vi "PosStrikerAnguloAttacker.vi"(8 "AnguloGol":dbl, 9 "atacando contra":bool, 10 "IA State":T1={"our_robots"=[], "enemy_robots"=[], "balls"=[], "geometry"={"line_width"=0, "field_length"=0, "field_width"=0, "boundary_width"=0, "referee_width"=0, "goal_width"=0, "goal_depth"=0, "goal_wall_width"=0, "center_circle_radius"=0, "defense_radius"=0, "defense_stretch"=0, "free_kick_from_defense_dist"=0, "penalty_spot_from_field_line_dist"=0, "penalty_line_from_spot_dist"=0}, "IA Judge"={"stage"="", "command"="", "our_goalie_id"=0.0, "enemy_goalie_id"=0.0, "command enum"=enum."Halt", "Time"=enum."Azul"}, "Received Timestamp"=timestamp(0 s since 1904-01-01), "Events"={"Touch"=FALSE, "Ball out"=FALSE, "id touch"=0.0, "Ball out of \nVision"=FALSE, "Ball inside \nGoalie area"=FALSE, "Robot not responding"=FALSE, "Robots responding status"=[1.0, 1.0, 1.0, 1.0, 1.0, 1.0], "Enemy Ball \nPossession"=FALSE, "Pass State"=FALSE, "id end of pass"=0.0, "Kick"=FALSE, "Id Possession"=0.0}, "Position"=[]}) -> (0 "YdoAttacker 2":dbl, 1 "AttackerPositive?":bool, 2 "theta final":dbl, 3 "XdoAttacker 2":dbl)   [LabVIEW 2016]
uses:
  Core/AI Input.ctl
  Core/AI Robot.ctl
  Intel/Functions Enum.ctl
  Intel/AttackerStates.ctl
  Core/AI Ball.ctl
  Core/Field Size.ctl
  Core/AI Judge.ctl
  Intel/Command Enum.ctl
  Events/Events.ctl
panel:
  in  "valor de theta 3":dbl
  in  "tamanho do intervalo 3":dbl
  in  "inicio do intervalo 3":dbl
  in  "fim do intervalo 3":dbl
  in  "Contador 4":dbl
  in  "Array 3":dbl[](array[numeric])=[0.0, 0.0, 0.0, 0.0, 0.0, 0.0]
  in  "valor de theta 2":dbl
  in  "tamanho do intervalo 2":dbl
  in  "inicio do intervalo 2":dbl
  in  "fim do intervalo 2":dbl
  in  "Contador 3":dbl
  in  "Array 2":dbl[](array[numeric])=[0.0, 0.0, 0.0, 0.0, 0.0, 0.0]
  in  "XdoAttacker":dbl
  in  "YdoAttacker":dbl
  in  "RobôsParaAnalisar":dbl[][](array[numeric])=[[99999.0, 99999.0], [99999.0, 99999.0], [99999.0, 99999.0], [99999.0, 99999.0], [99999.0, 99999.0], [99999.0, 99999.0], [99999.0, 99999.0]]
  in  "Contador":dbl
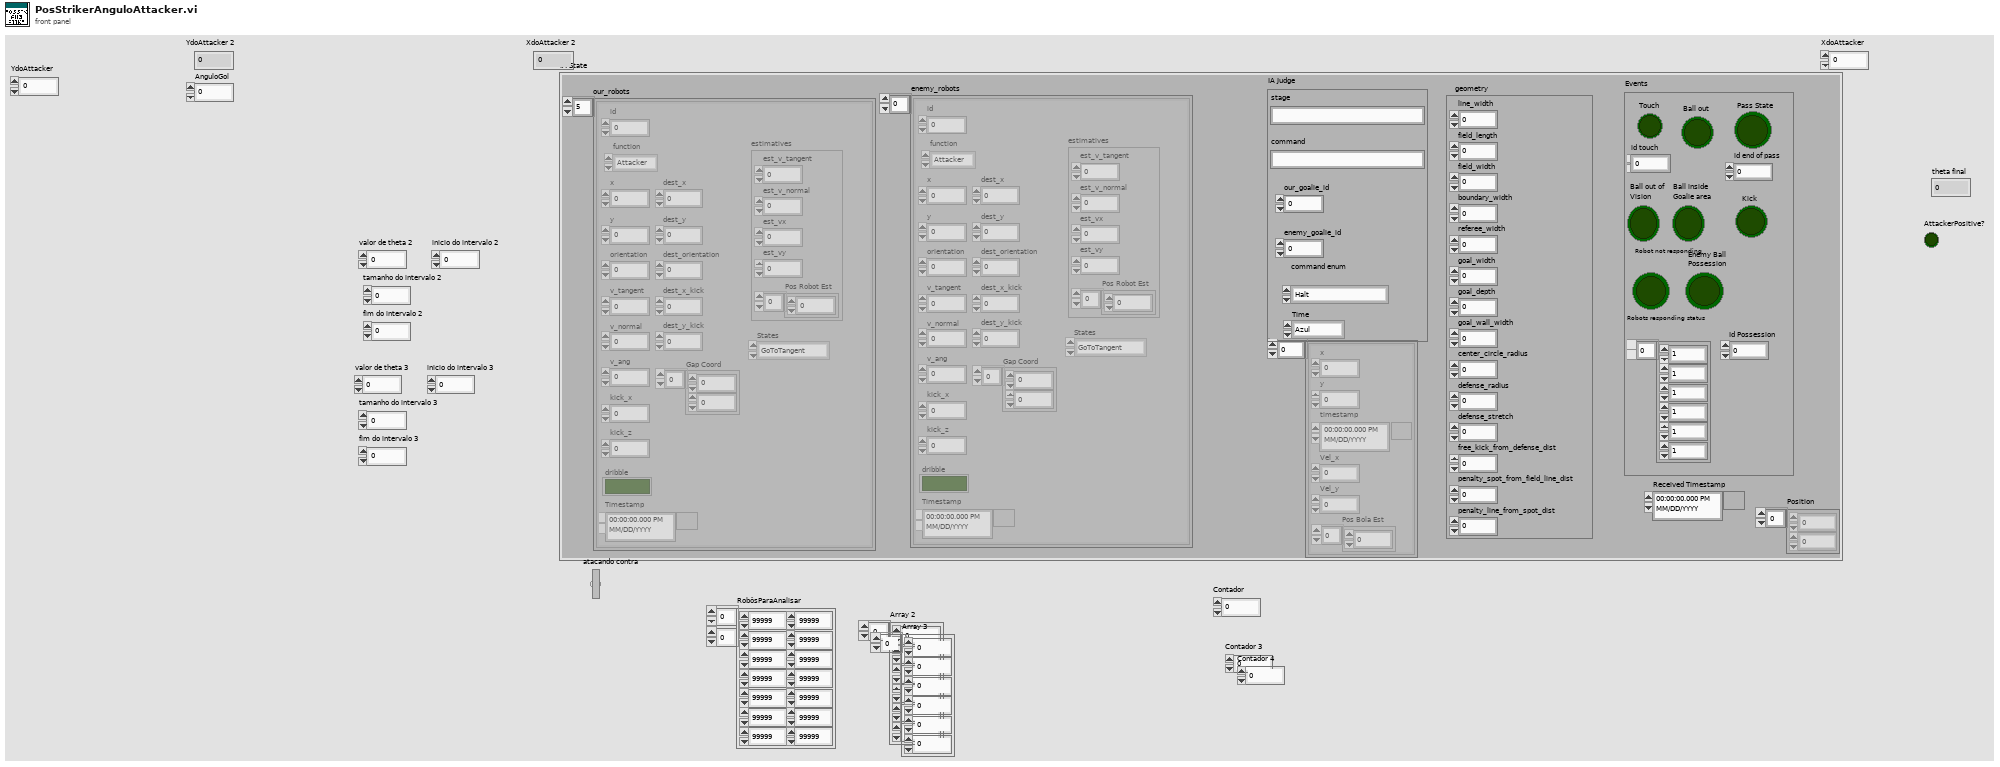
[diagram p1: front panel]
types:
  T1 = typedef "AI Input.ctl" = cluster{"our_robots":T2[], "enemy_robots":T2[], "balls":T5[], "geometry":T6, "IA Judge":T7, "Received Timestamp":timestamp, "Events":T9, "Position":dbl[]}
  T2 = typedef "AI Robot.ctl" = cluster{"id":u32, "function":T3, "x":dbl, "y":dbl, "orientation":dbl, "v_tangent":dbl, "v_normal":dbl, "v_ang":dbl, "kick_x":dbl, "kick_z":dbl, "dribble":bool, "Timestamp":timestamp, "dest_x":dbl, "dest_y":dbl, "dest_orientation":dbl, "estimatives":cluster{"est_v_tangent":dbl, "est_v_normal":dbl, "est_vx":dbl, "est_vy":dbl, "Pos Robot Est":dbl[]}, "dest_x_kick":dbl, "dest_y_kick":dbl, "Gap Coord":dbl[], "States":T4}
  T3 = typedef "Functions Enum.ctl" = enum16{"Attacker", "Goalie", "Defender", "Striker", "Goto 0", "Dummy", "Kicker", "ZigZag"}
  T4 = typedef "AttackerStates.ctl" = enum16{"Pass", "GoToTangent", "BallGetting", "GoToKick", ""}
  T5 = typedef "AI Ball.ctl" = cluster{"x":dbl, "y":dbl, "timestamp":timestamp, "Vel_x":dbl, "Vel_y":dbl, "Pos Bola Est":dbl[]}
  T6 = typedef "Field Size.ctl" = cluster{"line_width":u32, "field_length":u32, "field_width":u32, "boundary_width":u32, "referee_width":u32, "goal_width":u32, "goal_depth":u32, "goal_wall_width":u32, "center_circle_radius":u32, "defense_radius":u32, "defense_stretch":u32, "free_kick_from_defense_dist":u32, "penalty_spot_from_field_line_dist":u32, "penalty_line_from_spot_dist":u32}
  T7 = typedef "AI Judge.ctl" = cluster{"stage":string, "command":string, "our_goalie_id":dbl, "enemy_goalie_id":dbl, "command enum":T8, "Time":enum16{"Azul", "Amarelo"}}
  T8 = typedef "Command Enum.ctl" = enum16{"Halt", "Stop", "Force Start", "PKA Normal Start", "Prepare Kickoff Ally", "PKE Normal Start", "Prepare Kickoff Enemy", "Prepare Penalty Ally", "PPA Normal Start", "Prepare Penalty Enemy", "PPE Normal Start", "Direct Free Enemy", "Direct Free Ally", "Indirect Free Enemy", "Indirect Free Ally", "Timeout Enemy", "Timeout Ally", "Goal Enemy", "Goal Ally", "Ball Placement Enemy", "Ball Placement Ally", "Normal Half Time", "Extra Time Break", "Extra Half Time", "None"}
  T9 = typedef "Events.ctl" = cluster{"Touch":bool, "Ball out":bool, "id touch":dbl, "Ball out of \nVision":bool, "Ball inside \nGoalie area":bool, "Robot not responding":bool, "Robots responding status":dbl[], "Enemy Ball \nPossession":bool, "Pass State":bool, "id end of pass":dbl, "Kick":bool, "Id Possession":dbl}
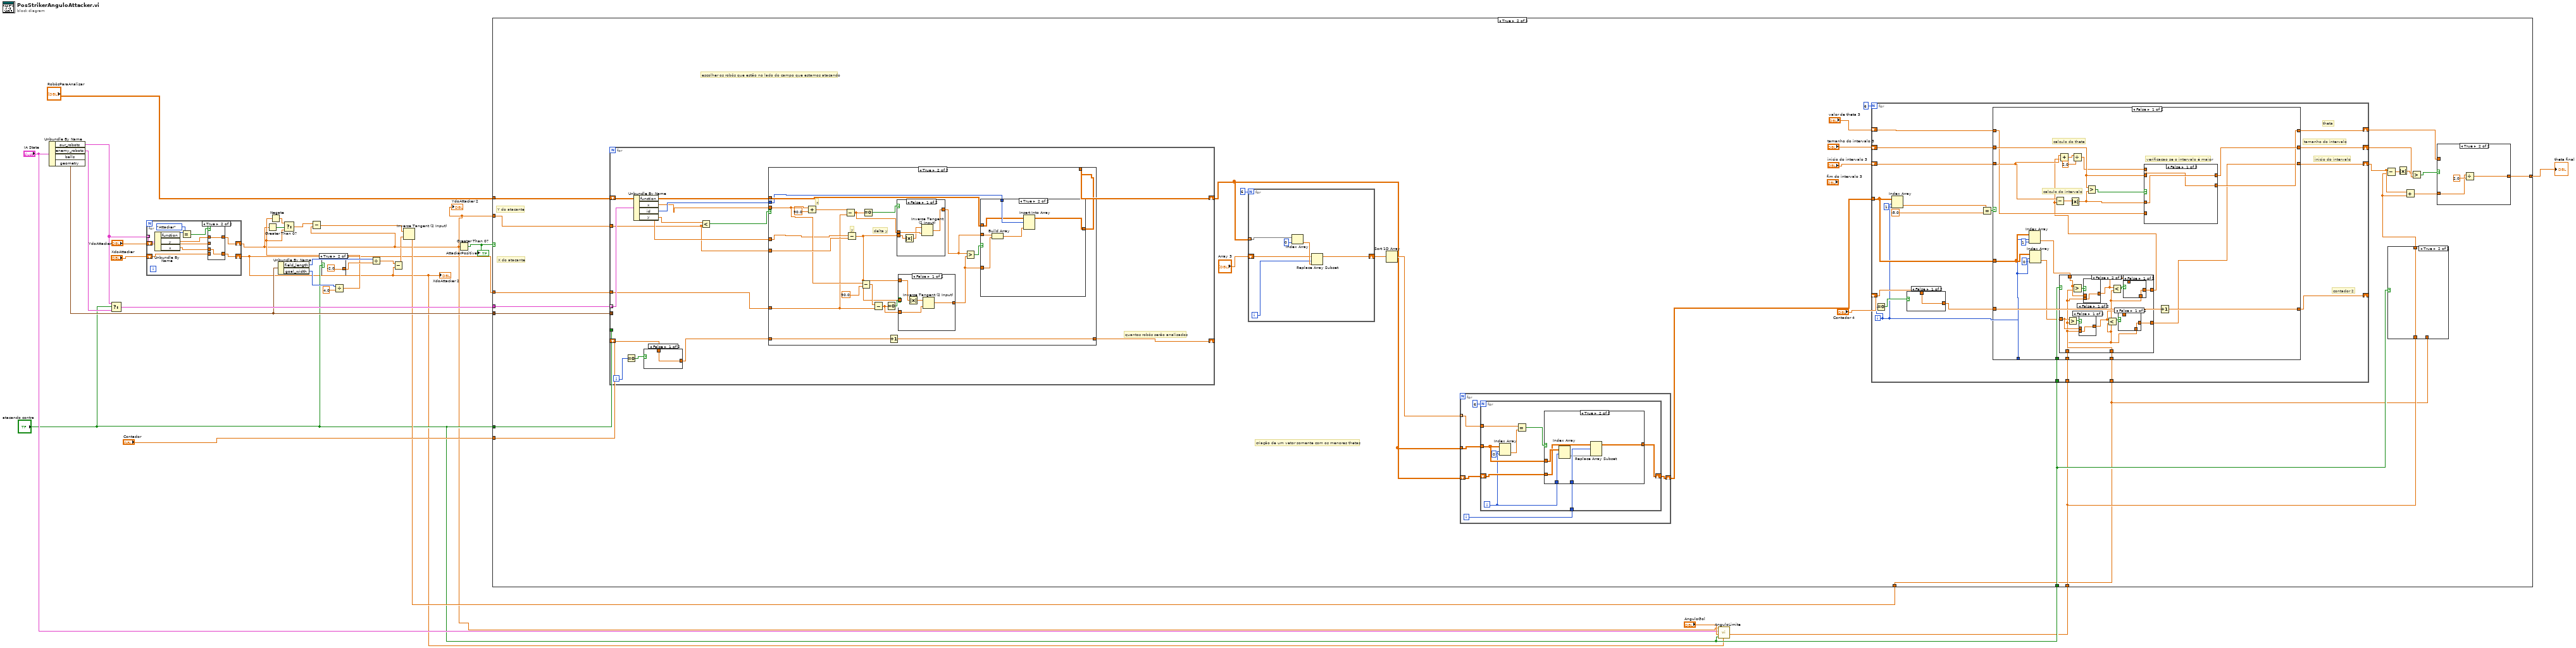
[diagram p0: block diagram]
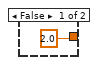
[diagram p2: hidden frame]
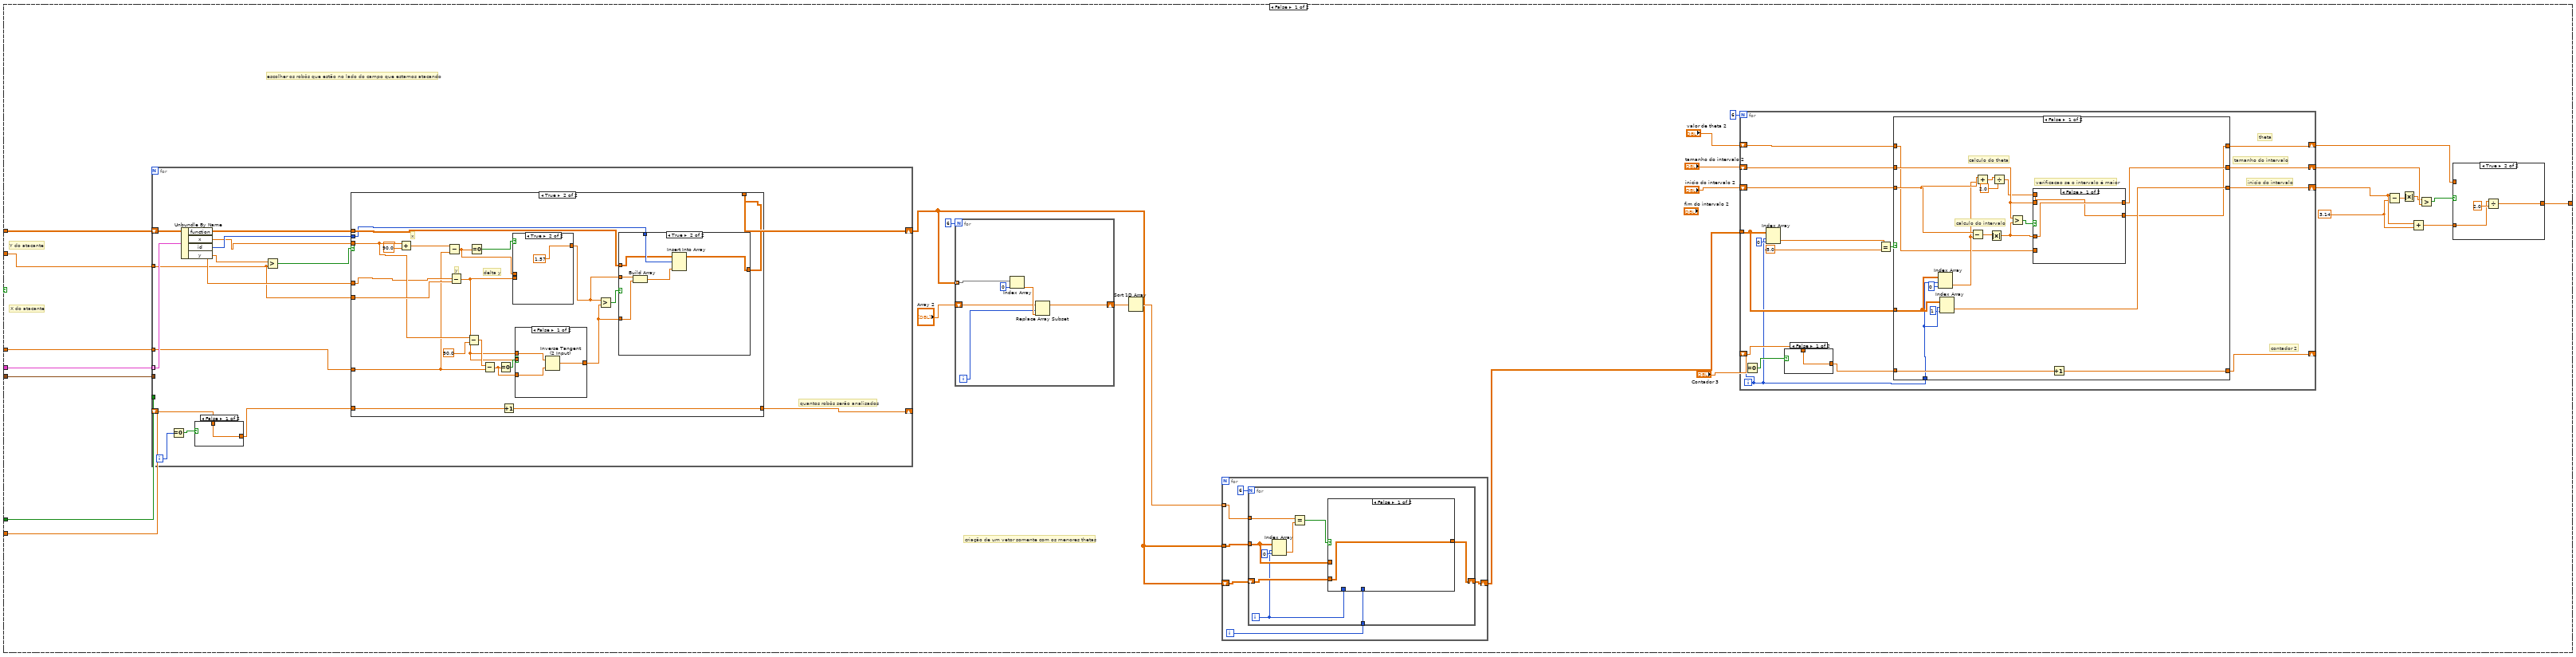
[diagram p3: hidden frame]
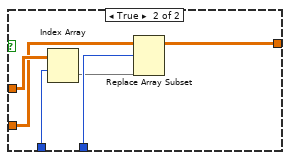
[diagram p5: hidden frame]
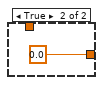
[diagram p6: hidden frame]
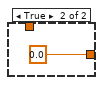
[diagram p9: hidden frame]
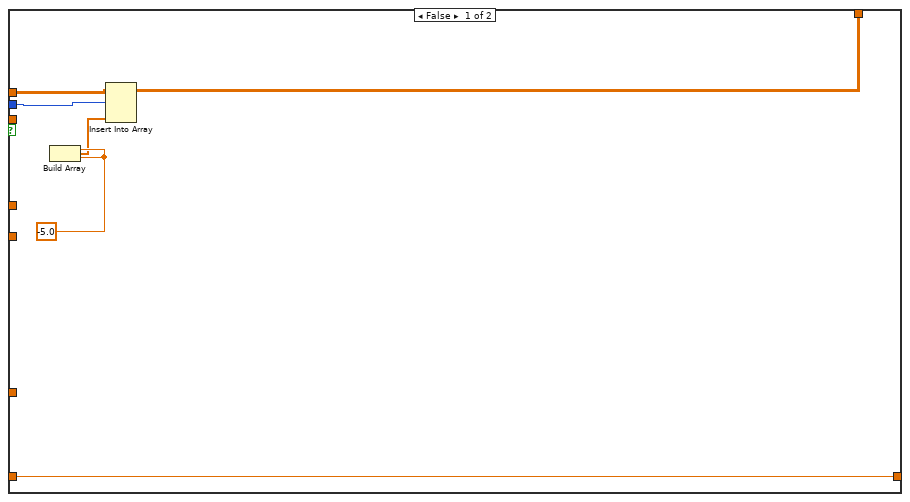
[diagram p10: hidden frame]
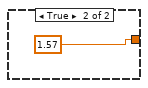
[diagram p11: hidden frame]
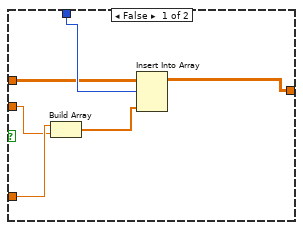
[diagram p12: hidden frame]
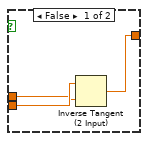
[diagram p13: hidden frame]
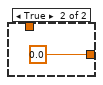
[diagram p17: hidden frame]
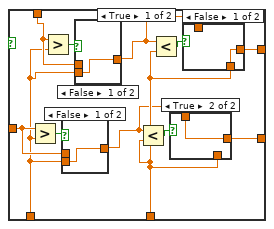
[diagram p18: hidden frame]
diagram:
  n1 = Unbundle By Name("IA State") -> ("our_robots"=w23:T2[], "enemy_robots"=w28:T2[], "geometry"=w14:T6)  [unwired: 1 out]
  n2 = Select(t=w23, s="atacando contra", f=w28) -> (s? t:f=w27:T2[])
  n3 = for {
    tunnel: w23 -> [w38] mode=indexing
    shift-right: [w33] -> w5
    shift-left: "YdoAttacker" -> [w32]
    shift-right: [w29] -> w1
    shift-left: "XdoAttacker" -> [w30]
    n4 = Unbundle By Name(w38) -> ("function"=w37:T3, "y"=w34:dbl, "x"=w31:dbl)
    n5 = Equal?(x=w37, y=Functions_Enum."Attacker") -> (x = y?=w35:bool)
    n6 = case shown="True" w35 {
      tunnel: w34 -> [_ w42]
      tunnel: [w40 w42] -> w33
      tunnel: w32 -> [w40 _]
      tunnel: w31 -> [_ w41]
      tunnel: w30 -> [w39 _]
      tunnel: [w39 w41] -> w29
      frame False {
      }
      frame True {
      }
    }
  }
  "YdoAttacker 2" <- w5
  "XdoAttacker 2" <- w1
  n7 = Greater Than 0?(x=w5) -> (x > 0?=w18:bool)
  n8 = Unbundle By Name(w14) -> ("field_length"=w19:u32, "goal_width"=w12:u32)
  n9 = case shown="True" "atacando contra" {
    tunnel: [2.0 ("y") -2.0 ("y")] -> w15
    frame False {
    }
    frame True {
    }
  }
  n10 = Divide(x=w12, y=4.0) -> (x/y=w11:dbl)
  n11 = Negate(x=w11) -> (-x=w17:dbl)
  n12 = Select(t=w17, s=w18, f=w11) -> (s? t:f=w4:dbl)
  n13 = Subtract(x=w4, y=w5) -> (x-y=w16:dbl)
  n14 = Divide(x=w19, y=w15) -> (x/y=w2:dbl)
  n15 = Subtract(x=w2, y=w1) -> (x-y=w3:dbl)
  n16 = Inverse Tangent (2 Input)(1:w3, 2:w16) -> (0:w10:dbl)
  n17 = Greater Than 0?(x=w5) -> (x > 0?=w20:bool)
  "AttackerPositive?" <- w20
  n18 = call "AnguloLimite.vi"("XdoAttacker"=w1, "atacando contra"="atacando contra", "AnguloGol"="AnguloGol", "IA State"="IA State", "YdoAttacker"=w5) -> ("Angulo Limite"=w6:dbl)  [unwired: 6 in]
  n19 = case shown="True" w20 {
    tunnel: w27 -> [w71 w241]
    tunnel: "atacando contra" -> [w70 w240]
    tunnel: "Contador" -> [w69 w239]
    tunnel: "RobôsParaAnalisar" -> [w68 w238]
    tunnel: w14 -> [w67 w237]
    tunnel: [w53 w223] -> w24
    tunnel: w5 -> [w46 w217]
    tunnel: w1 -> [w45 w216]
    tunnel: w10 -> [_ w212]
    tunnel: "atacando contra" -> [_ w215]
    tunnel: w6 -> [_ w214]
    frame False {
      w48 = 3.14 ("y")
      # "X do atacante"
      # "Y do atacante"
      # "criação de um vetor somente com os menores thetas"
      # "escolher os robôs que estão no lado do campo que estamos atacando"
      n20 = for {
        tunnel: w71 -> [w162] mode=indexing
        tunnel: w70 -> [_]
        shift-right: [w154] -> w57
        shift-left: w68 -> [w161]
        shift-right: [w155] -> _
        shift-left: w69 -> [w157]
        tunnel: w67 -> [_]
        tunnel: w46 -> [w150]
        tunnel: w45 -> [w149]
        i -> [w158]
        # "quantos robôs serão analisados"
        n21 = Equal To 0?(x=w158) -> (x = 0?=w159:bool)
        n22 = Unbundle By Name(w162) -> ("x"=w153:dbl, "id"=w160:u32, "y"=w152:dbl)  [unwired: 1 out]
        n23 = case shown="False" w159 {
          tunnel: w157 -> [w163 _]
          tunnel: [w163 0.0] -> w156
          frame False {
          }
          frame True {
          }
        }
        n24 = Greater?(x=w152, y=w150) -> (0:w151:bool)
        n25 = case shown="True" w151 {
          tunnel: w161 -> [w169 w189]
          tunnel: w160 -> [w168 w188]
          tunnel: w153 -> [_ w179]
          tunnel: w152 -> [_ w178]
          tunnel: w156 -> [w170 w190]
          tunnel: [w170 w191] -> w155
          tunnel: [w165 w187] -> w154
          tunnel: w150 -> [_ w180]
          tunnel: w149 -> [_ w176]
          frame False {
            w167 = -5.0 ("element")
            n26 = Build Array(w167, w167) -> (w166:dbl[])
            n27 = Insert Into Array(array=w169, index (row)=w168, new element=w166) -> (w165:dbl[][])  [unwired: 1 in]
          }
          frame True {
            # "delta y"
            # "y"
            # "x"
            n28 = Add(x=w179, y=90.0) -> (x+y=w177:dbl)
            n29 = Subtract(x=w177, y=w176) -> (x-y=w174:dbl)
            n30 = Subtract(x=w178, y=w180) -> (x-y=w171:dbl)
            n31 = Subtract(x=w179, y=90.0) -> (x-y=w184:dbl)
            n32 = Equal To 0?(x=w174) -> (x = 0?=w175:bool)
            n33 = Subtract(x=w184, y=w176) -> (x-y=w172:dbl)
            n34 = Equal To 0?(x=w172) -> (x = 0?=w173:bool)
            n35 = Increment(x=w190) -> (x+1=w191:dbl)
            n36 = case shown="True" w175 {
              tunnel: [w209 1.57] -> w182
              tunnel: w171 -> [w210 _]
              tunnel: w174 -> [w208 _]
              frame False {
                n37 = Inverse Tangent (2 Input)(1:w208, 2:w210) -> (0:w209:dbl)
              }
              frame True {
              }
            }
            n38 = case shown="False" w173 {
              tunnel: [w194 1.57] -> w181
              tunnel: w171 -> [_ _]
              tunnel: w172 -> [w193 _]
              tunnel: w171 -> [w192 _]
              frame False {
                n39 = Inverse Tangent (2 Input)(1:w193, 2:w192) -> (0:w194:dbl)
              }
              frame True {
              }
            }
            n40 = Greater?(x=w182, y=w181) -> (0:w183:bool)
            n41 = case shown="True" w183 {
              tunnel: w189 -> [w198 w204]
              tunnel: w188 -> [w200 w207]
              tunnel: w182 -> [w197 w205]
              tunnel: w181 -> [w199 w203]
              tunnel: [w196 w202] -> w187
              frame False {
                n42 = Build Array(w199, w197) -> (w201:dbl[])
                n43 = Insert Into Array(array=w198, index (row)=w200, new element=w201) -> (w196:dbl[][])  [unwired: 1 in]
              }
              frame True {
                n44 = Build Array(w205, w203) -> (w206:dbl[])
                n45 = Insert Into Array(array=w204, index (row)=w207, new element=w206) -> (w202:dbl[][])  [unwired: 1 in]
              }
            }
          }
        }
      }
      n46 = for {
        N: 6 -> [_]
        tunnel: w57 -> [w103] mode=indexing
        shift-right: [w98] -> w59
        shift-left: "Array 2" -> [w99]
        i -> [w100]
        n47 = Index Array(array=w103, index=0) -> (element=w101:dbl)
        n48 = Replace Array Subset(array=w99, new element=w101, index=w100) -> (w98:dbl[])
      }
      n49 = Sort 1D Array(array=w59) -> (sorted array=w58:dbl[])
      n50 = for {
        tunnel: w58 -> [w78] mode=indexing
        tunnel: w57 -> [w80]
        shift-right: [w76] -> w56
        shift-left: w57 -> [w79]
        i -> [w77]
        n51 = for {
          N: 6 -> [_]
          tunnel: w80 -> [w86]
          shift-right: [w82] -> w76
          shift-left: w79 -> [w85]
          tunnel: w78 -> [w88]
          tunnel: w77 -> [w83]
          i -> [w84]
          n52 = Index Array(array=w86, index (row)=w84, index (col)=0 ("disabled index (col)")) -> (element=w89:dbl)
          n53 = Equal?(x=w88, y=w89) -> (x = y?=w87:bool)
          n54 = case shown="False" w87 {
            tunnel: w86 -> [_ w97]
            tunnel: w85 -> [w91 w93]
            tunnel: w84 -> [_ w96]
            tunnel: w83 -> [_ w95]
            tunnel: [w91 w92] -> w82
            frame False {
            }
            frame True {
              n55 = Index Array(array=w97, index (row)=w96) -> (element=w94:dbl[])  [unwired: 1 in]
              n56 = Replace Array Subset(array=w93, new element=w94, index (row)=w95) -> (w92:dbl[][])  [unwired: 1 in]
            }
          }
        }
      }
      n57 = for {
        N: 6 -> [_]
        tunnel: w56 -> [w105]
        shift-right: [w114] -> w52
        shift-left: "valor de theta 2" -> [w115]
        shift-right: [w112] -> w55
        shift-left: "tamanho do intervalo 2" -> [w113]
        shift-right: [w110] -> w49
        shift-left: "inicio do intervalo 2" -> [w111]
        shift-right: [w106] -> _
        shift-left: "Contador 3" -> [w108]
        i -> [w104]
        # "contador 2"
        # "inicio do intervalo"
        # "tamanho do intervalo"
        # "theta"
        n58 = Equal To 0?(x=w104) -> (x = 0?=w109:bool)
        n59 = Index Array(array=w105, index (row)=w104, index (col)=0 ("disabled index (col)")) -> (element=w117:dbl)
        n60 = case shown="False" w109 {
          tunnel: w108 -> [w120 _]
          tunnel: [w120 0.0] -> w107
          frame False {
          }
          frame True {
          }
        }
        n61 = Equal?(x=w117, y=-5.0) -> (x = y?=w118:bool)
        n62 = case shown="False" w118 {
          tunnel: w115 -> [w122 w148]
          tunnel: [w123 w148] -> w114
          tunnel: w113 -> [w127 w147]
          tunnel: [w126 w147] -> w112
          tunnel: w111 -> [w140 w146]
          tunnel: [w135 w146] -> w110
          tunnel: w107 -> [w138 w145]
          tunnel: [w139 w145] -> w106
          tunnel: w105 -> [w137 _]
          tunnel: w104 -> [w136 _]
          frame False {
            # "calculo do theta"
            # "calculo do intervalo"
            # "verificacao se o intervalo é maior"
            n63 = Index Array(array=w137, index (row)=w136, index (col)=0 ("disabled index (col)")) -> (element=w131:dbl)
            n64 = Index Array(array=w137, index (row)=w136, index (col)=1 ("disabled index (col)")) -> (element=w135:dbl)
            n65 = Subtract(x=w140, y=w131) -> (x-y=w132:dbl)
            n66 = Add(x=w140, y=w131) -> (x+y=w130:dbl)
            n67 = Absolute Value(x=w132) -> (abs(x)=w125:dbl)
            n68 = Divide(x=w130, y=2.0) -> (x/y=w124:dbl)
            n69 = Greater?(x=w127, y=w125) -> (0:w128:bool)
            n70 = case shown="False" w128 {
              tunnel: w127 -> [_ w144]
              tunnel: [w142 w144] -> w126
              tunnel: w125 -> [w142 _]
              tunnel: w122 -> [_ w143]
              tunnel: w124 -> [w141 _]
              tunnel: [w141 w143] -> w123
              frame False {
              }
              frame True {
              }
            }
            n71 = Increment(x=w138) -> (x+1=w139:dbl)
          }
          frame True {
          }
        }
      }
      n72 = Subtract(x=w49, y=w48) -> (x-y=w51:dbl)
      n73 = Absolute Value(x=w51) -> (abs(x)=w50:dbl)
      n74 = Add(x=w49, y=w48) -> (x+y=w47:dbl)
      n75 = Greater?(x=w50, y=w55) -> (0:w54:bool)
      n76 = case shown="True" w54 {
        tunnel: [w72 w74] -> w53
        tunnel: w52 -> [w72 _]
        tunnel: w47 -> [_ w73]
        frame False {
        }
        frame True {
          n77 = Divide(x=w73, y=2.0) -> (x/y=w74:dbl)
        }
      }
    }
    frame True {
      # "X do atacante"
      # "Y do atacante"
      # "criação de um vetor somente com os menores thetas"
      # "escolher os robôs que estão no lado do campo que estamos atacando"
      n78 = for {
        tunnel: w241 -> [w382] mode=indexing
        tunnel: w240 -> [_]
        shift-right: [w374] -> w227
        shift-left: w238 -> [w381]
        shift-right: [w375] -> _
        shift-left: w239 -> [w377]
        tunnel: w237 -> [_]
        tunnel: w217 -> [w370]
        tunnel: w216 -> [w369]
        i -> [w378]
        # "quantos robôs serão analisados"
        n79 = Equal To 0?(x=w378) -> (x = 0?=w379:bool)
        n80 = Unbundle By Name(w382) -> ("x"=w373:dbl, "id"=w380:u32, "y"=w372:dbl)  [unwired: 1 out]
        n81 = case shown="False" w379 {
          tunnel: w377 -> [w383 _]
          tunnel: [w383 0.0] -> w376
          frame False {
          }
          frame True {
          }
        }
        n82 = Less?(x=w372, y=w370) -> (x < y?=w371:bool)
        n83 = case shown="True" w371 {
          tunnel: w381 -> [w389 w409]
          tunnel: w380 -> [w388 w408]
          tunnel: w373 -> [_ w399]
          tunnel: w372 -> [_ w398]
          tunnel: w376 -> [w390 w410]
          tunnel: [w390 w411] -> w375
          tunnel: [w385 w407] -> w374
          tunnel: w370 -> [_ w400]
          tunnel: w369 -> [_ w396]
          frame False {
            w387 = -5.0 ("element")
            n84 = Build Array(w387, w387) -> (w386:dbl[])
            n85 = Insert Into Array(array=w389, index (row)=w388, new element=w386) -> (w385:dbl[][])  [unwired: 1 in]
          }
          frame True {
            # "delta y"
            # "y"
            # "x"
            n86 = Add(x=w399, y=90.0) -> (x+y=w397:dbl)
            n87 = Subtract(x=w397, y=w396) -> (x-y=w394:dbl)
            n88 = Subtract(x=w398, y=w400) -> (x-y=w391:dbl)
            n89 = Subtract(x=w399, y=90.0) -> (x-y=w404:dbl)
            n90 = Equal To 0?(x=w394) -> (x = 0?=w395:bool)
            n91 = Subtract(x=w404, y=w396) -> (x-y=w392:dbl)
            n92 = Equal To 0?(x=w392) -> (x = 0?=w393:bool)
            n93 = Increment(x=w410) -> (x+1=w411:dbl)
            n94 = case shown="False" w395 {
              tunnel: [w432 1.57] -> w402
              tunnel: w391 -> [w430 _]
              tunnel: w394 -> [w431 _]
              frame False {
                n95 = Absolute Value(x=w430) -> (abs(x)=w429:dbl)
                n96 = Inverse Tangent (2 Input)(1:w431, 2:w429) -> (0:w432:dbl)
              }
              frame True {
              }
            }
            n97 = case shown="False" w393 {
              tunnel: [w415 1.57] -> w401
              tunnel: w391 -> [_ _]
              tunnel: w392 -> [w414 _]
              tunnel: w391 -> [w412 _]
              frame False {
                n98 = Absolute Value(x=w412) -> (abs(x)=w413:dbl)
                n99 = Inverse Tangent (2 Input)(1:w414, 2:w413) -> (0:w415:dbl)
              }
              frame True {
              }
            }
            n100 = Greater?(x=w402, y=w401) -> (0:w403:bool)
            n101 = case shown="True" w403 {
              tunnel: w409 -> [w419 w425]
              tunnel: w408 -> [w421 w428]
              tunnel: w402 -> [w418 w426]
              tunnel: w401 -> [w420 w424]
              tunnel: [w417 w423] -> w407
              frame False {
                n102 = Build Array(w420, w418) -> (w422:dbl[])
                n103 = Insert Into Array(array=w419, index (row)=w421, new element=w422) -> (w417:dbl[][])  [unwired: 1 in]
              }
              frame True {
                n104 = Build Array(w426, w424) -> (w427:dbl[])
                n105 = Insert Into Array(array=w425, index (row)=w428, new element=w427) -> (w423:dbl[][])  [unwired: 1 in]
              }
            }
          }
        }
      }
      n106 = for {
        N: 6 -> [_]
        tunnel: w227 -> [w275] mode=indexing
        shift-right: [w270] -> w229
        shift-left: "Array 3" -> [w271]
        i -> [w272]
        n107 = Index Array(array=w275, index=0) -> (element=w273:dbl)
        n108 = Replace Array Subset(array=w271, new element=w273, index=w272) -> (w270:dbl[])
      }
      n109 = Sort 1D Array(array=w229) -> (sorted array=w228:dbl[])
      n110 = for {
        tunnel: w228 -> [w250] mode=indexing
        tunnel: w227 -> [w252]
        shift-right: [w248] -> w226
        shift-left: w227 -> [w251]
        i -> [w249]
        n111 = for {
          N: 6 -> [_]
          tunnel: w252 -> [w258]
          shift-right: [w254] -> w248
          shift-left: w251 -> [w257]
          tunnel: w250 -> [w260]
          tunnel: w249 -> [w255]
          i -> [w256]
          n112 = Index Array(array=w258, index (row)=w256, index (col)=0 ("disabled index (col)")) -> (element=w261:dbl)
          n113 = Equal?(x=w260, y=w261) -> (x = y?=w259:bool)
          n114 = case shown="True" w259 {
            tunnel: w258 -> [_ w269]
            tunnel: w257 -> [w263 w265]
            tunnel: w256 -> [_ w268]
            tunnel: w255 -> [_ w267]
            tunnel: [w263 w264] -> w254
            frame False {
            }
            frame True {
              n115 = Index Array(array=w269, index (row)=w268) -> (element=w266:dbl[])  [unwired: 1 in]
              n116 = Replace Array Subset(array=w265, new element=w266, index (row)=w267) -> (w264:dbl[][])  [unwired: 1 in]
            }
          }
        }
      }
      n117 = for {
        N: 6 -> [_]
        tunnel: w226 -> [w280]
        shift-right: [w289] -> w222
        shift-left: "valor de theta 3" -> [w290]
        shift-right: [w287] -> w225
        shift-left: "tamanho do intervalo 3" -> [w288]
        shift-right: [w285] -> w219
        shift-left: "inicio do intervalo 3" -> [w286]
        shift-right: [w281] -> _
        shift-left: "Contador 4" -> [w283]
        tunnel: w215 -> [w278]
        tunnel: w214 -> [w277]
        tunnel: w212 -> [w276]
        i -> [w279]
        # "contador 2"
        # "inicio do intervalo"
        # "tamanho do intervalo"
        # "theta"
        n118 = Equal To 0?(x=w279) -> (x = 0?=w284:bool)
        n119 = Index Array(array=w280, index (row)=w279, index (col)=1 ("disabled index (col)")) -> (element=w292:dbl)
        n120 = case shown="False" w284 {
          tunnel: w283 -> [w295 _]
          tunnel: [w295 0.0] -> w282
          frame False {
          }
          frame True {
          }
        }
        n121 = Equal?(x=w292, y=-5.0) -> (x = y?=w293:bool)
        n122 = case shown="False" w293 {
          tunnel: w290 -> [w304 w368]
          tunnel: [w305 w368] -> w289
          tunnel: w288 -> [w309 w367]
          tunnel: [w308 w367] -> w287
          tunnel: w286 -> [w320 w366]
          tunnel: [w297 w366] -> w285
          tunnel: w282 -> [w318 w365]
          tunnel: [w319 w365] -> w281
          tunnel: w280 -> [w317 _]
          tunnel: w279 -> [w316 _]
          tunnel: w278 -> [w303 _]
          tunnel: w277 -> [w302 _]
          tunnel: w276 -> [w301 _]
          frame False {
            # "calculo do theta"
            # "calculo do intervalo"
            # "verificacao se o intervalo é maior"
            n123 = Index Array(array=w317, index (row)=w316, index (col)=1 ("disabled index (col)")) -> (element=w300:dbl)
            n124 = Index Array(array=w317, index (row)=w316, index (col)=0 ("disabled index (col)")) -> (element=w298:dbl)
            n125 = case shown="False" w303 {
              tunnel: w302 -> [w324 w342]
              tunnel: w300 -> [w331 w351]
              tunnel: w301 -> [w323 w343]
              tunnel: [w329 w349] -> w299
              tunnel: w298 -> [w325 w345]
              tunnel: [w322 w344] -> w297
              frame True {
                n126 = Greater?(x=w325, y=w324) -> (0:w327:bool)
                n127 = Greater?(x=w331, y=w324) -> (0:w332:bool)
                n128 = case shown="False" w327 {
                  tunnel: [w335 w336] -> w321
                  tunnel: w325 -> [_ w336]
                  tunnel: w324 -> [w335 _]
                  frame False {
                  }
                  frame True {
                  }
                }
                n129 = case shown="False" w332 {
                  tunnel: [w339 w340] -> w328
                  tunnel: w331 -> [_ w340]
                  tunnel: w324 -> [w339 _]
                  frame False {
                  }
                  frame True {
                  }
                }
                n130 = Less?(x=w321, y=w323) -> (x < y?=w326:bool)
                n131 = Less?(x=w328, y=w323) -> (x < y?=w330:bool)
                n132 = case shown="True" w326 {
                  tunnel: [w333 w334] -> w322
                  tunnel: w321 -> [_ w334]
                  tunnel: w323 -> [w333 _]
                  frame False {
                  }
                  frame True {
                  }
                }
                n133 = case shown="False" w330 {
                  tunnel: [w337 w338] -> w329
                  tunnel: w328 -> [_ w338]
                  tunnel: w323 -> [w337 _]
                  frame False {
                  }
                  frame True {
                  }
                }
              }
              frame False {
                n134 = Greater?(x=w345, y=w343) -> (0:w347:bool)
                n135 = Greater?(x=w351, y=w343) -> (0:w352:bool)
                n136 = case shown="False" w347 {
                  tunnel: [w355 w356] -> w341
                  tunnel: w345 -> [_ w356]
                  tunnel: w343 -> [w355 _]
                  frame False {
                  }
                  frame True {
                  }
                }
                n137 = case shown="False" w352 {
                  tunnel: [w359 w360] -> w348
                  tunnel: w351 -> [_ w360]
                  tunnel: w343 -> [w359 _]
                  frame False {
                  }
                  frame True {
                  }
                }
                n138 = Less?(x=w341, y=w342) -> (x < y?=w346:bool)
                n139 = Less?(x=w348, y=w342) -> (x < y?=w350:bool)
                n140 = case shown="False" w346 {
                  tunnel: [w353 w354] -> w344
                  tunnel: w341 -> [_ w354]
                  tunnel: w342 -> [w353 _]
                  frame False {
                  }
                  frame True {
                  }
                }
                n141 = case shown="False" w350 {
                  tunnel: [w357 w358] -> w349
                  tunnel: w348 -> [_ w358]
                  tunnel: w342 -> [w357 _]
                  frame False {
                  }
                  frame True {
                  }
                }
              }
            }
            n142 = Subtract(x=w320, y=w299) -> (x-y=w313:dbl)
            n143 = Add(x=w320, y=w299) -> (x+y=w312:dbl)
            n144 = Absolute Value(x=w313) -> (abs(x)=w307:dbl)
            n145 = Divide(x=w312, y=2.0) -> (x/y=w306:dbl)
            n146 = Greater?(x=w309, y=w307) -> (0:w310:bool)
            n147 = case shown="False" w310 {
              tunnel: w309 -> [_ w364]
              tunnel: [w362 w364] -> w308
              tunnel: w307 -> [w362 _]
              tunnel: w304 -> [_ w363]
              tunnel: w306 -> [w361 _]
              tunnel: [w361 w363] -> w305
              frame False {
              }
              frame True {
              }
            }
            n148 = Increment(x=w318) -> (x+1=w319:dbl)
          }
          frame True {
          }
        }
      }
      n149 = case shown="True" w215 {
        tunnel: w214 -> [_ w243]
        tunnel: [w242 w243] -> w213
        tunnel: w212 -> [w242 _]
        frame False {
        }
        frame True {
        }
      }
      n150 = Subtract(x=w219, y=w213) -> (x-y=w221:dbl)
      n151 = Absolute Value(x=w221) -> (abs(x)=w220:dbl)
      n152 = Add(x=w219, y=w213) -> (x+y=w218:dbl)
      n153 = Greater?(x=w220, y=w225) -> (0:w224:bool)
      n154 = case shown="True" w224 {
        tunnel: [w244 w246] -> w223
        tunnel: w222 -> [w244 _]
        tunnel: w218 -> [_ w245]
        frame False {
        }
        frame True {
          n155 = Divide(x=w245, y=2.0) -> (x/y=w246:dbl)
        }
      }
    }
  }
  "theta final" <- w24
